vi "filter.vi"(10 "data_input":dbl[](array[numeric])) -> (2 "appended array":dbl[](array[numeric]))   [LabVIEW 2020]
uses:
  <vilib>/ptbypt/NI_PtbyPt.lvlib
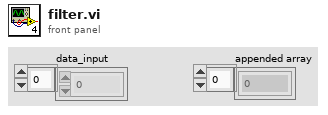
[diagram p1: front panel]
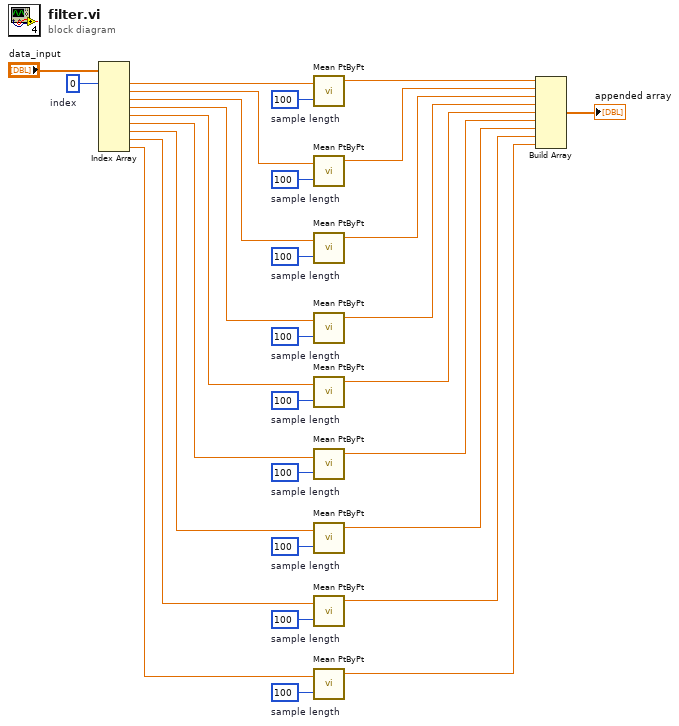
[diagram p0: block diagram]
diagram:
  w13 = 100  # sample length
  w14 = 100  # sample length
  w30 = 100  # sample length
  w29 = 100  # sample length
  w28 = 100  # sample length
  w27 = 100  # sample length
  w26 = 100  # sample length
  w25 = 100  # sample length
  w24 = 100  # sample length
  w22 = 0  # index
  n1 = Index Array(array="data_input", index #1=w22) -> (element #1=w23:dbl, element #2=w20:dbl, element #3=w19:dbl, element #4=w18:dbl, element #5=w17:dbl, element #6=w16:dbl, element #7=w15:dbl, element #8=w12:dbl, element #9=w11:dbl)  [unwired: 8 in]
  n2 = call <vilib>:"Mean PtByPt.vi"("x"=w23, "sample length"=w24) -> ("mean"=w10:dbl)  [unwired: 2 in, 1 out]
  n3 = call <vilib>:"Mean PtByPt.vi"("x"=w20, "sample length"=w25) -> ("mean"=w9:dbl)  [unwired: 2 in, 1 out]
  n4 = call <vilib>:"Mean PtByPt.vi"("x"=w19, "sample length"=w26) -> ("mean"=w8:dbl)  [unwired: 2 in, 1 out]
  n5 = call <vilib>:"Mean PtByPt.vi"("x"=w18, "sample length"=w27) -> ("mean"=w7:dbl)  [unwired: 2 in, 1 out]
  n6 = call <vilib>:"Mean PtByPt.vi"("x"=w17, "sample length"=w28) -> ("mean"=w6:dbl)  [unwired: 2 in, 1 out]
  n7 = call <vilib>:"Mean PtByPt.vi"("x"=w16, "sample length"=w29) -> ("mean"=w5:dbl)  [unwired: 2 in, 1 out]
  n8 = call <vilib>:"Mean PtByPt.vi"("x"=w15, "sample length"=w30) -> ("mean"=w4:dbl)  [unwired: 2 in, 1 out]
  n9 = call <vilib>:"Mean PtByPt.vi"("x"=w12, "sample length"=w14) -> ("mean"=w3:dbl)  [unwired: 2 in, 1 out]
  n10 = call <vilib>:"Mean PtByPt.vi"("x"=w11, "sample length"=w13) -> ("mean"=w2:dbl)  [unwired: 2 in, 1 out]
  n11 = Build Array(w10, w9, w8, w7, w6, w5, w4, w3, w2) -> (→"appended array":dbl[])
